vi "Write CAN Frames.vi"(7 "CAN Channel":u16=1, 8 "error in (no error)":errorcluster, 10 "Frames":T1[](array[typedef]) {"type" items=["CAN Data"=0, "CAN Remote"=1, "CAN Bus Error"=2, "CAN 2.0 Data"=8, "CAN FD Data"=16, "CAN FD+BRS Data"=24, "J1939 Data"=192, "Delay"=224, "Log Trigger"=225, "Start Trigger"=226]; "payload" format="%x"; "timestamp" format="%<%.7X\n%x>T"; "identifier" format="%x"}, 11 "Read Write BLF in":refnum<class "Read Write BLF.lvclass">) -> (0 "error out":errorcluster, 3 "Read Write BLF out":refnum<class "Read Write BLF.lvclass">)   [LabVIEW 2015, in "Read Write BLF.lvclass"]
doc: "This VI will write N <B>CAN frames</B> to a BLF File.\n\n-------------\nBrian Hoover (Hooovahh)"
uses:
  Read Write BLF.lvclass
  Controls/Cluster - CAN Frame.ctl
  Controls/Enum - CAN Data Type.ctl
  Read Write BLF.lvclass/Read Write BLF.ctl
  Set Measurement Start Time.vi
  SubVIs/GetBinlogdllpath.vi
  <vilib>/Utility/error.llb/Error Cluster From Error Code.vi
  <vilib>/Utility/file.llb/Application Directory.vi
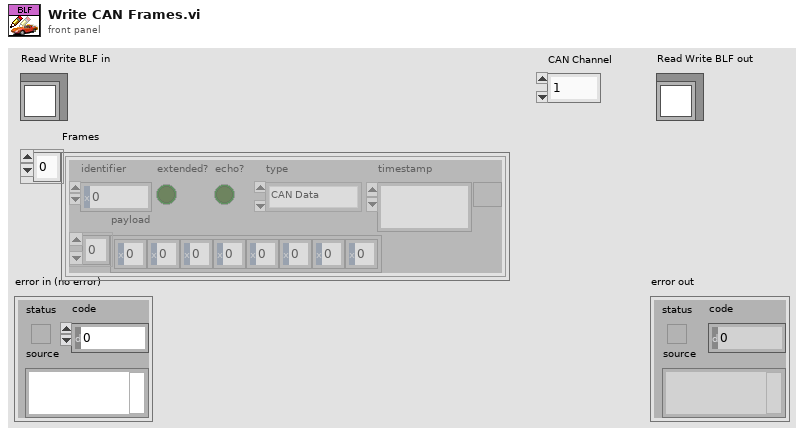
[diagram p1: front panel]
types:
  T1 = typedef "Read Write BLF.lvclass/Cluster - CAN Frame.ctl" = cluster{"timestamp":timestamp, "payload":u8[], "identifier":u32, "extended?":bool, "echo?":bool, "type":T2}
  T2 = typedef "Read Write BLF.lvclass/Enum - CAN Data Type.ctl" = u8
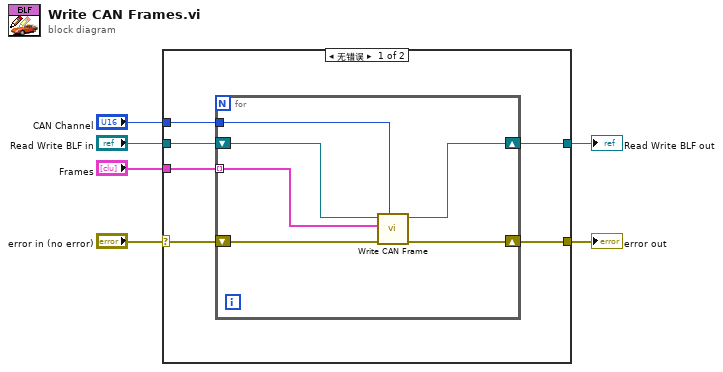
[diagram p0: block diagram]
diagram:
  n1 = case shown="无错误" "error in (no error)" {
    selector: "error in (no error)" -> [w9 w20]
    tunnel: [w8 w20] -> w5
    tunnel: [w10 w19] -> w3
    tunnel: "Read Write BLF in" -> [w11 w19]
    tunnel: "Frames" -> [w12 _]
    tunnel: "CAN Channel" -> [w7 _]
    frame No Error {
      n2 = for {
        tunnel: w12 -> [w16] mode=indexing
        shift-right: [w17] -> w10
        shift-left: w11 -> [w18]
        shift-right: [w14] -> w8
        shift-left: w9 -> [w15]
        tunnel: w7 -> [w13]
        n3 = call "Write CAN Frame.vi"("CAN Channel"=w13, "error in (no error)"=w15, "CAN Frame"=w16, "BLF File In"=w18) -> ("error out"=w14:errorcluster, "BLF File Out"=w17:refnum<class "Read Write BLF.lvclass">)  [unwired: 6 in]
      }
    }
    frame Error {
    }
  }
  "error out" <- w5
  "Read Write BLF out" <- w3
